vi "Idle_Timer.vi"(8 "error in (no error)":errorcluster) -> (0 "error out":errorcluster)   [LabVIEW 2020]
uses:
  Controls/Idle_Timer.ctl
  Controls/Idle_Timer_disp.ctl
panel:
  in  "Exit":bool
  in  "Save":bool
  in  "Idle Timer":T1={"OP10"=0.2, "OP20"=0.2, "OP30"=0.2, "OP40"=0.2, "OP50"=0.2, "OP60"=0.2} {"OP60" min=0.1 max=9999999.0; "OP50" min=0.1 max=9999999.0; "OP40" min=0.1 max=9999999.0; "OP30" min=0.1 max=9999999.0; "OP20" min=0.1 max=9999999.0; "OP10" min=0.1 max=9999999.0}
  # "Idle Timer"
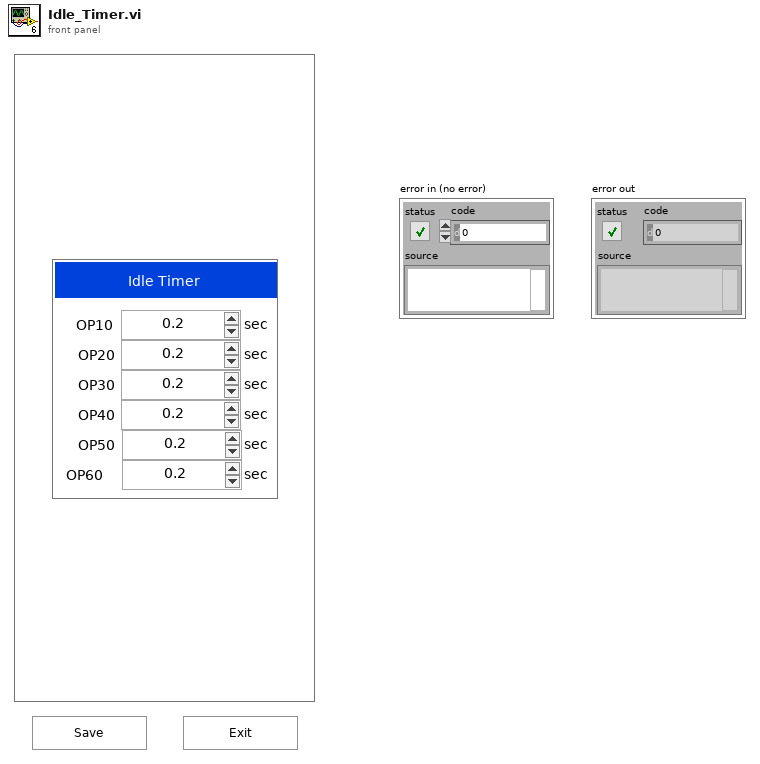
[diagram p1: front panel]
types:
  T1 = typedef "Idle_Timer.ctl" = cluster{"OP10":T2, "OP20":T2, "OP30":T2, "OP40":T2, "OP50":T2, "OP60":T2}
  T2 = typedef "Idle_Timer_disp.ctl" = dbl
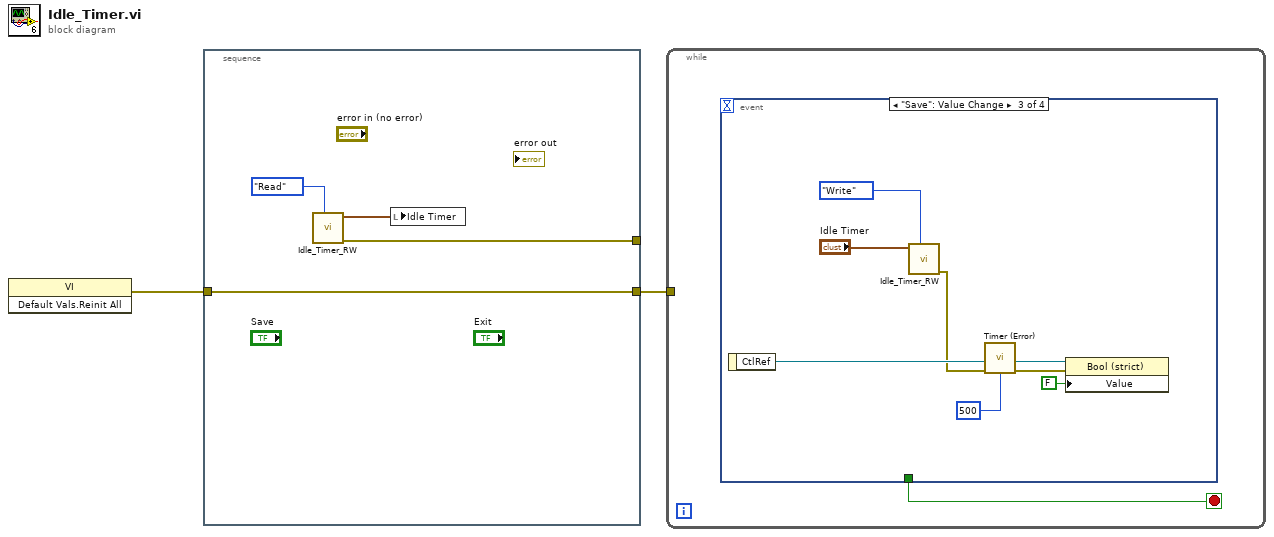
[diagram p0: block diagram]
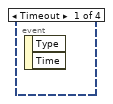
[diagram p2: hidden frame]
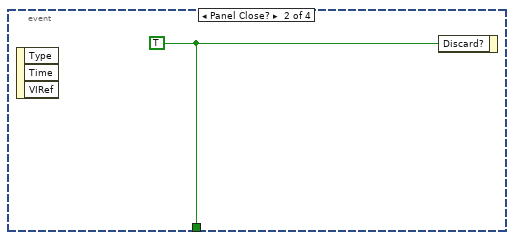
[diagram p3: hidden frame]
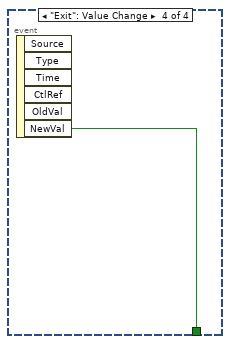
[diagram p4: hidden frame]
diagram:
  n1 = invoke class="VI" method="Default Vals.Reinit All"() -> (error out=w2:errorcluster)  [unwired: 3 in, 2 out]
  n2 = stacked-sequence {
    tunnel: [w6] -> w1
    tunnel: w2 -> [w6]
    tunnel: [w3] -> _
    frame #0 {
      n3 = call "Idle_Timer_RW.vi"("R/W"=enum16{"Write", "Read"}."Read") -> ("error out"=w3:errorcluster, "Idle Timer Out"=w4:T1)  [unwired: 9 in]
      n4 = local write "Idle Timer"(w4) -> ()
    }
  }
  n5 = while {
    tunnel: w1 -> [_]
    stop <- w7 stop-if-true
    n6 = event shown="[2] \"Save\": Value Change" {
      selector: _ -> [_ _ _ _]
      dyn-events: _ -> [_ _ _ _]
      timeout: _ -> [_ _ _ _]
      tunnel: [_ w8 _ w16] -> w7
      event Timeout {
        n7 = event-data() -> ()  [unwired: 1 in, 2 out]
      }
      event Panel Close? {
        w8 = TRUE ("Discard?")
        n8 = event-data() -> ()  [unwired: 1 in, 3 out]
        n9 = event-data("Discard?"=w8) -> ()  [unwired: 1 in, 1 out]
      }
      event "Save": Value Change {
        n10 = event-data() -> ("CtlRef"=w13:refnum<vi>)  [unwired: 1 in]
        n11 = call "Idle_Timer_RW.vi"("R/W"=enum16{"Write", "Read"}."Write", "Idle Timer In"="Idle Timer") -> ("error out"=w11:errorcluster)  [unwired: 8 in, 1 out]
        n12 = call <userlib>:"Timer (Error).vi"("error in (no error)"=w11, "milliseconds to wait"=u32 500) -> ("error out"=w9:errorcluster)  [unwired: 13 in]
        n13 = property class="Bool (strict)"(reference=w13, error in=w9, "Value"=FALSE ("Value (Signaling)")) -> ()  [unwired: 2 out]
      }
      event "Exit": Value Change {
        n14 = event-data() -> ("NewVal"=w16:bool)  [unwired: 1 in, 5 out]
      }
    }
  }
